vi "数据处理直接插入整合 (子VI).vi"   [LabVIEW 2016, in "数据传输系统.lvlib"]
types:
  T1 = cluster{"PH":string[][], "CODCr":string[][], "氨氮":string[][], "CODMn":string[][], "总氮":string[][], "总磷":string[][], "电导率":string[][], "水温":string[][], "DO":string[][], "浊度":string[][], "叶绿素":string[][], "藻密度":string[][], "铜":string[][], "盐度":string[][], "水位":string[][], "流速":string[][], "瞬时流量":string[][], "累积流量":string[][], "亚硝酸盐":string[][], "硫化物":string[][], "ORP":string[][], "铅":string[][], "ïÓ":string[][], "锌":string[][], "镍":string[][], "锰":string[][], "汞":string[][], "气温":string[][], "气压":string[][], "风速":string[][], "风向":string[][], "盐度 2":string[][], "磷酸盐":string[][], "硝氮":string[][], "氟化物":string[][], "挥发酚":string[][], "氯化物":string[][]}
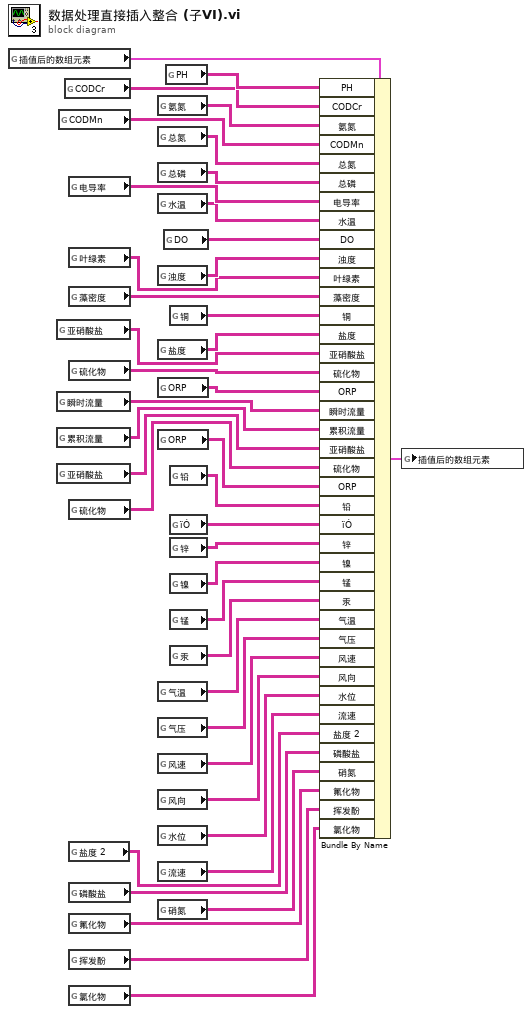
[diagram p0: block diagram]
diagram:
  n1 = global read "插值后的新数组.vi" "插值后的数组元素"() -> (w28:T1)
  n2 = global read "全局 所有参数.vi" "亚硝酸盐"() -> (w25:string[][])
  n3 = global read "全局 所有参数.vi" "瞬时流量"() -> (w23:string[][])
  n4 = global read "全局 所有参数.vi" "累积流量"() -> (w22:string[][])
  n5 = global read "全局 所有参数.vi" "亚硝酸盐"() -> (w21:string[][])
  n6 = global read "全局 所有参数.vi" "CODMn"() -> (w39:string[][])
  n7 = global read "全局 所有参数.vi" "CODCr"() -> (w41:string[][])
  n8 = global read "全局 所有参数.vi" "电导率"() -> (w36:string[][])
  n9 = global read "全局 所有参数.vi" "叶绿素"() -> (w32:string[][])
  n10 = global read "全局 所有参数.vi" "藻密度"() -> (w31:string[][])
  n11 = global read "全局 所有参数.vi" "硫化物"() -> (w26:string[][])
  n12 = global read "全局 所有参数.vi" "硫化物"() -> (w20:string[][])
  n13 = global read "全局 所有参数.vi" "盐度 2"() -> (w6:string[][])
  n14 = global read "全局 所有参数.vi" "磷酸盐"() -> (w5:string[][])
  n15 = global read "全局 所有参数.vi" "氟化物"() -> (w3:string[][])
  n16 = global read "全局 所有参数.vi" "挥发酚"() -> (w2:string[][])
  n17 = global read "全局 所有参数.vi" "氯化物"() -> (w1:string[][])
  n18 = global read "全局 所有参数.vi" "氨氮"() -> (w40:string[][])
  n19 = global read "全局 所有参数.vi" "总氮"() -> (w38:string[][])
  n20 = global read "全局 所有参数.vi" "总磷"() -> (w37:string[][])
  n21 = global read "全局 所有参数.vi" "水温"() -> (w35:string[][])
  n22 = global read "全局 所有参数.vi" "浊度"() -> (w33:string[][])
  n23 = global read "全局 所有参数.vi" "盐度"() -> (w29:string[][])
  n24 = global read "全局 所有参数.vi" "ORP"() -> (w27:string[][])
  n25 = global read "全局 所有参数.vi" "ORP"() -> (w19:string[][])
  n26 = global read "全局 所有参数.vi" "气温"() -> (w12:string[][])
  n27 = global read "全局 所有参数.vi" "气压"() -> (w11:string[][])
  n28 = global read "全局 所有参数.vi" "风速"() -> (w10:string[][])
  n29 = global read "全局 所有参数.vi" "风向"() -> (w9:string[][])
  n30 = global read "全局 所有参数.vi" "水位"() -> (w8:string[][])
  n31 = global read "全局 所有参数.vi" "流速"() -> (w7:string[][])
  n32 = global read "全局 所有参数.vi" "硝氮"() -> (w4:string[][])
  n33 = global read "全局 所有参数.vi" "DO"() -> (w34:string[][])
  n34 = global read "全局 所有参数.vi" "PH"() -> (w42:string[][])
  n35 = global read "全局 所有参数.vi" "铜"() -> (w30:string[][])
  n36 = global read "全局 所有参数.vi" "铅"() -> (w18:string[][])
  n37 = global read "全局 所有参数.vi" "ïÓ"() -> (w17:string[][])
  n38 = global read "全局 所有参数.vi" "锌"() -> (w16:string[][])
  n39 = global read "全局 所有参数.vi" "镍"() -> (w15:string[][])
  n40 = global read "全局 所有参数.vi" "锰"() -> (w14:string[][])
  n41 = global read "全局 所有参数.vi" "汞"() -> (w13:string[][])
  n42 = Bundle By Name(cluster=w28, "PH"=w42, "CODCr"=w41, "氨氮"=w40, "CODMn"=w39, "总氮"=w38, "总磷"=w37, "电导率"=w36, "水温"=w35, "DO"=w34, "浊度"=w33, "叶绿素"=w32, "藻密度"=w31, "铜"=w30, "盐度"=w29, "亚硝酸盐"=w25, "硫化物"=w26, "ORP"=w27, "瞬时流量"=w23, "累积流量"=w22, "亚硝酸盐"=w21, "硫化物"=w20, "ORP"=w19, "铅"=w18, "ïÓ"=w17, "锌"=w16, "镍"=w15, "锰"=w14, "汞"=w13, "气温"=w12, "气压"=w11, "风速"=w10, "风向"=w9, "水位"=w8, "流速"=w7, "盐度 2"=w6, "磷酸盐"=w5, "硝氮"=w4, "氟化物"=w3, "挥发酚"=w2, "氯化物"=w1) -> (w24:T1)
  n43 = global write "插值后的新数组.vi" "插值后的数组元素"(w24) -> ()
